vi "retrieveConfiguration.vi"(8 "error in (no error)":errorcluster, 10 "dataName":string, 11 "WindowsTarget in":refnum<class "WindowsTarget.lvclass">) -> (0 "error out":errorcluster, 2 "dataValueFromFile":string, 3 "WindowsTarget out":refnum<class "WindowsTarget.lvclass">)   [LabVIEW 2015, in "WindowsTarget.lvclass"]
doc: "Retrieves the configuration data from the file associated with dataName."
uses:
  WindowsTarget.lvclass
  ComponentTemplateCore/ComponentModel/ComponentModelDT/ConfigurationFileReaderDT/ConfigurationFileReaderDT.lvclass
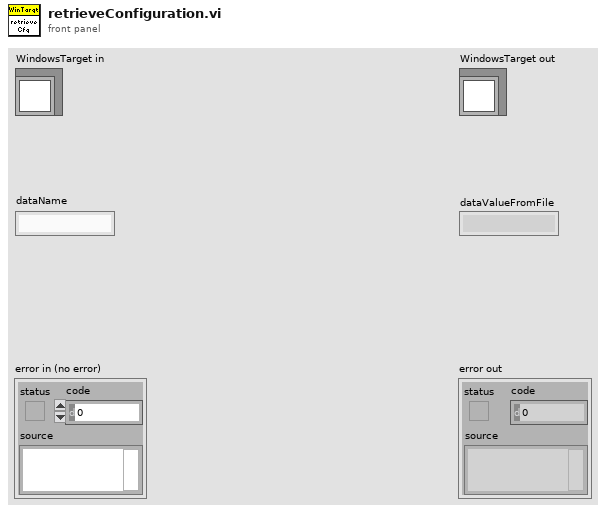
[diagram p1: front panel]
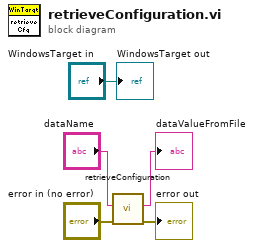
[diagram p0: block diagram]
diagram:
  n1 = call "retrieveConfiguration.vi"("error in (no error)"="error in (no error)", "dataName"="dataName") -> ("error out"=→"error out":errorcluster, "dataValueFromFile"=→"dataValueFromFile":string)  [unwired: 7 in, 1 out]
  "WindowsTarget out" <- "WindowsTarget in"
